vi "Close Instrument.vi"(8 "error in (no error)":errorcluster, 11 "instrument.PPMS2 in":refnum<class "instrument.PPMS2.lvclass">) -> (0 "error out":errorcluster, 3 "instrument.PPMS2 out":refnum<class "instrument.PPMS2.lvclass">)   [LabVIEW 2016, in "instrument.PPMS2.lvclass"]
uses:
  instrument.PPMS2.lvclass
  instrument.PPMS2.lvclass/instrument.PPMS2.ctl
  C:/Users/patrick/Documents/GitHub/PPMS-Monitor-and-Control/lvsrc/drivers/QDInstrument_LabView/QDInstrument.dll
  drivers/QDInstrument_LabView/QDInstrument.dll
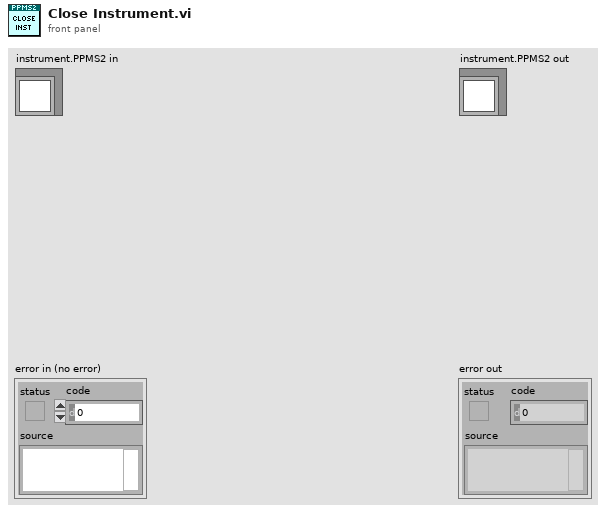
[diagram p1: front panel]
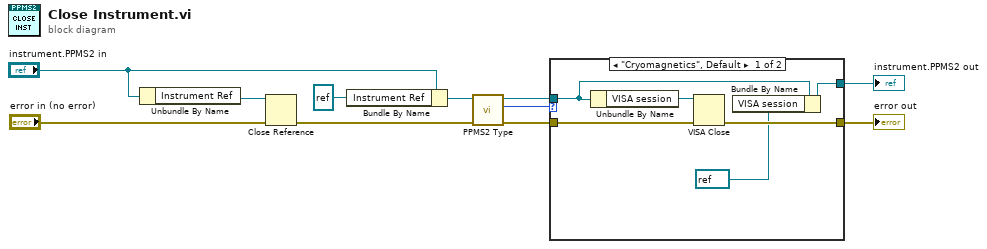
[diagram p0: block diagram]
diagram:
  n1 = Unbundle By Name("instrument.PPMS2 in") -> ("Instrument Ref"=w11:refnum<k24>)
  n2 = Close Reference(reference=w11, error in (no error)="error in (no error)") -> (error out=w3:errorcluster)
  n3 = Bundle By Name(cluster="instrument.PPMS2 in", "Instrument Ref"=refnum<k24> refnum) -> (w8:refnum<class "instrument.PPMS2.lvclass">)
  n4 = call "PPMS2 Type.vi"("error in (no error)"=w3, "instrument.PPMS2 in"=w8) -> ("error out"=w2:errorcluster, "PPMS \"Type\""=w7:enum16{"Cryomagnetics", "QD only"}, "instrument.PPMS2 out"=w5:refnum<class "instrument.PPMS2.lvclass">)  [unwired: 7 in]
  n5 = case shown="\"Cryomagnetics\", Default" w7 {
    tunnel: [w13 w19] -> w6
    tunnel: w5 -> [w14 w19]
    tunnel: w2 -> [w17 w18]
    tunnel: [w16 w18] -> w1
    frame "Cryomagnetics", Default {
      n6 = Unbundle By Name(w14) -> ("VISA session"=w15:refnum<visa-resource-name>)
      n7 = VISA Close(VISA resource name=w15, error in (no error)=w17) -> (error out=w16:errorcluster)
      n8 = Bundle By Name(cluster=w14, "VISA session"=refnum<visa-resource-name> refnum ("Cryomagnetics.VISA session")) -> (w13:refnum<class "instrument.PPMS2.lvclass">)
    }
    frame "QD only" {
    }
  }
  "error out" <- w1
  "instrument.PPMS2 out" <- w6
